vi "Main.vi"() -> ()   [LabVIEW 2013]
uses:
  Classes/My API/Post.ctl
  Classes/My API/My API.lvclass
panel:
  out "Create Post id":i32
  out "Post fetched":T1
  in  "Post to create":T1={"id"=0, "userId"=123, "title"="New post title", "body"="New post content"}
  # "Web Service Client Example"
  # "1. Get a specific item from the web service"
  # "2. Add a new item to the web service"
  # "Fill in the cluster below ignoring the \"id\" field"
  # "Copyright (c) 2017, JKI, all rights reserved!"
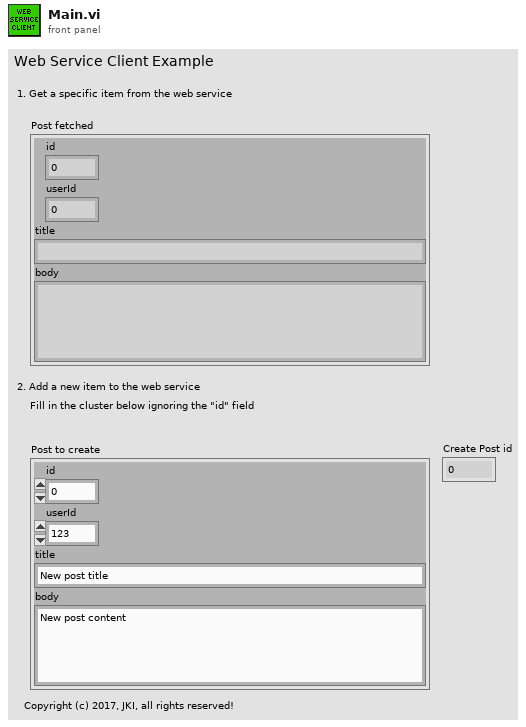
[diagram p1: front panel]
types:
  T1 = typedef "My API.lvclass/Post.ctl" = cluster{"id":i32, "userId":i32, "title":string, "body":string}
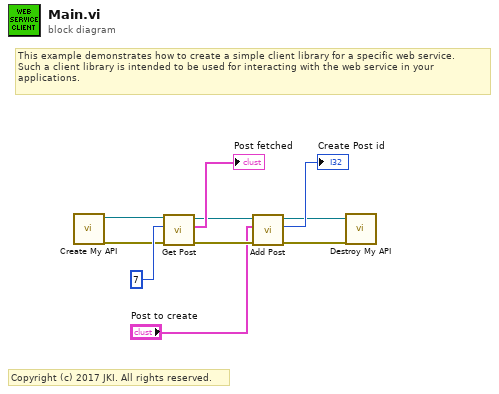
[diagram p0: block diagram]
diagram:
  # "This example demonstrates how to create a simple client library for a specific web service.\nSuch a client library is intended to be used for interacting with the web service in your\napplications."
  # "Copyright (c) 2017 JKI. All rights reserved."
  n1 = call "Create My API.vi"() -> ("error out"=w7:errorcluster, "My API out"=w8:refnum<class "My API.lvclass">)  [unwired: 10 in]
  n2 = call-dynamic "Get Post.vi"("error in (no error)"=w7, "id"=7, "My API in"=w8) -> ("error out"=w5:errorcluster, "Post"=→"Post fetched":T1, "My API out"=w6:refnum<class "My API.lvclass">)  [unwired: 6 in]
  n3 = call-dynamic "Add Post.vi"("error in (no error)"=w5, "Post"="Post to create", "My API in"=w6) -> ("error out"=w2:errorcluster, "id"=→"Create Post id":i32, "My API out"=w1:refnum<class "My API.lvclass">)  [unwired: 6 in]
  n4 = call-dynamic "Destroy My API.vi"("error in (no error)"=w2, "My API in"=w1) -> ()  [unwired: 9 in, 1 out]
